vi "Main Archive and FTP 4_0.vi"() -> ()   [LabVIEW 2011]
doc: "FILE Archive & FTP is a software used to handle the file management of remote field sites using the HTI Data Logger or ATR series acoustic equipment that generates *.RAT and *.ATL files. The software monitors a specific folder on the local machine that the HTI equipment has been set up to move completed files of these types into. All other file types are ignored. The software continues to scan this file until a new file is added to the directory, on the addition of a file the NODE ARCHIVE & FTP software moves the file into an Archive directory (and if specified into a redundant Archive directory) then creates a *.ZIP version of the file and retains a copy of it in the Archive directory as well. All Zip files are then copied to a specified FTP host.\n\nNODE ARCHIVE & FTP will not try and move files for the last five minutes of an hour, or for the first five to ten minutes of the hour (based on CPU time). This is to allow the HTI hardware time to move all files at the top of the hour and avoid conflict. During the rest of the hour the software will continue to scan for new files. At any time a user can force a scan or FTP move by selecting the Manual Force FTP button or the Manual Archive Files button.\n\nNODE ARCHIVE & FTP creates an .INI file and a .CSV file in the programs application directory. The .INI file retains the last values of the file directory and FTP credentials used. The .CSV retains a history of *.ZIP files moved to the FTP and the status of their move, if there were errors or not. NODE ARCHIVE & FTP will continue to try and send the file to the FTP host until that file has completed the process with no errors. DO NOT remove or edit the .CSV file or the software will try and move all files up to the FTP again and will slow down the FTP Host."
uses:
  <vilib>/Utility/error.llb/DialogType.ctl
  <vilib>/Utility/sysdir.llb/System Directory Type.ctl
  Controls/FTP Credintials.ctl
  Controls/File Management.ctl
  Controls/File Path directories.ctl
  Controls/Ping address and email notify.ctl
panel:
  in  "ShutDown 2":bool
  in  "File type Cover 2":bool
  in  "Manual Archive 2":bool
  out "Email Notification Cluster":T1={"Mail Server"="", "Return Address"="", "Email User Name"="", "Password"="", "Ping Address 1"="10.0.0.40", "Ping Address 2"="google.com", "Ping Address FTP Host"="web1026.ixwebhosting.com", "Ping address 1"=FALSE, "Ping address 2"=FALSE, "Ping FTP Host"=FALSE}
  in  "shutting down closeout":bool
  in  "Time DaY":timestamp
  in  "Top level Tabs":T2(tab)
  in  "Auto Archive":bool
  in  "Auto FTP":bool
  in  "FTP Creds":T3 {"FTP Timeout (S)" min=0 max=300 step=1}
  in  "SITE ID":string="Site Not Configured" caption="Site ID:"
  in  "File Management":T4
  in  "Manual FTP":bool
  out "Archive in progress":bool caption="Archive"
  out "Status FTP move":bool caption="FTP"
  in  "Manual Archive":bool
  in  "File output directories":T5={"Archive Location"=path "", "Archive Location 2"=path "<Not A Path>", "OutPut Path"=path "", "Directory(s) To Scan Files"=[]}
  in  "Ping FTP Host":bool
  in  "Ping on Address 2":bool
  in  "Ping on Address 1":bool
  out "Response 2":bool
  in  "AddressNode2":string="www.google.com" caption="Ping Address for 2"
  out "FTP Host\nResponse":bool
  out "Response 1":bool
  in  "recipients":string[](array[string])=["nmswyers@gmail.com"] caption="Errors & Warnings Email Recipients"
  in  "Addresshost":string="50.6.185.144" caption="Ping Address of FTP"
  in  "AddressNode 1":string="10.0.0.40" caption="Ping Address for 1"
  out "Elapsed Time (H)":dbl caption="Time since Last File \nSize Check (H)" format="%#_3f"
  # "D\nI\nR\nE\nC\nT\nO\nR\nY\n\nS\nE\nT"
  # "FTP\n\nSETUP"
  # "FILE \n\nHANDLE\n\nMETHODS"
  # "File Handling Method"
  # "Addresses to Ping"
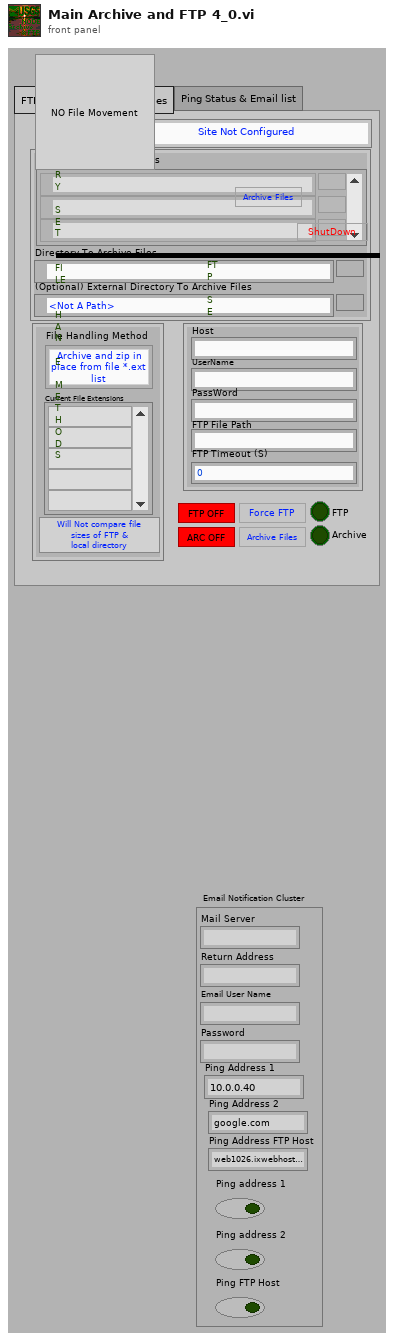
[diagram p1: front panel]
types:
  T1 = typedef "Ping address and email notify.ctl" = cluster{"Mail Server":string, "Return Address":string, "Email User Name":string, "Password":string, "Ping Address 1":string, "Ping Address 2":string, "Ping Address FTP Host":string, "Ping address 1":bool, "Ping address 2":bool, "Ping FTP Host":bool}
  T2 = enum32{"FTP Connection & Directories", "Ping Status & Email list"}
  T3 = typedef "FTP Credintials.ctl" = cluster{"Host":string, "UserName":string, "PassWord":string, "FTP File Path":string, "FTP Timeout (S)":i32, "Active or Passive":bool, "ASCII or Binary":bool}
  T4 = typedef "File Management.ctl" = cluster{"Comp File Size":bool, "File Handle Method":enum16{"Archive and zip in place from file *.ext list", "Archive and zip ALL file Types to archive directory", "Archive and zip to archive directory from file *.ext list", "Perform no file management"}, "file extention list":string[]}
  T5 = typedef "File Path directories.ctl" = cluster{"Archive Location":path, "Archive Location 2":path, "OutPut Path":path, "Directory(s) To Scan Files":path[]}
  T6 = enum16{"Archive and zip in place from file *.ext list", "Archive and zip ALL file Types to archive directory", "Archive and zip to archive directory from file *.ext list", "Perform no file management"}
  T7 = typedef "DialogType.ctl" = u16
  T8 = enum8{"Enabled", "Disabled", "Disabled and Grayed Out"}
  T9 = enum32{"invalid app kind", "Development System", "Run Time System", "Student Edition", "Embedded LabVIEW", "Evaluation", "Custom"}
  T10 = typedef "System Directory Type.ctl" = i32
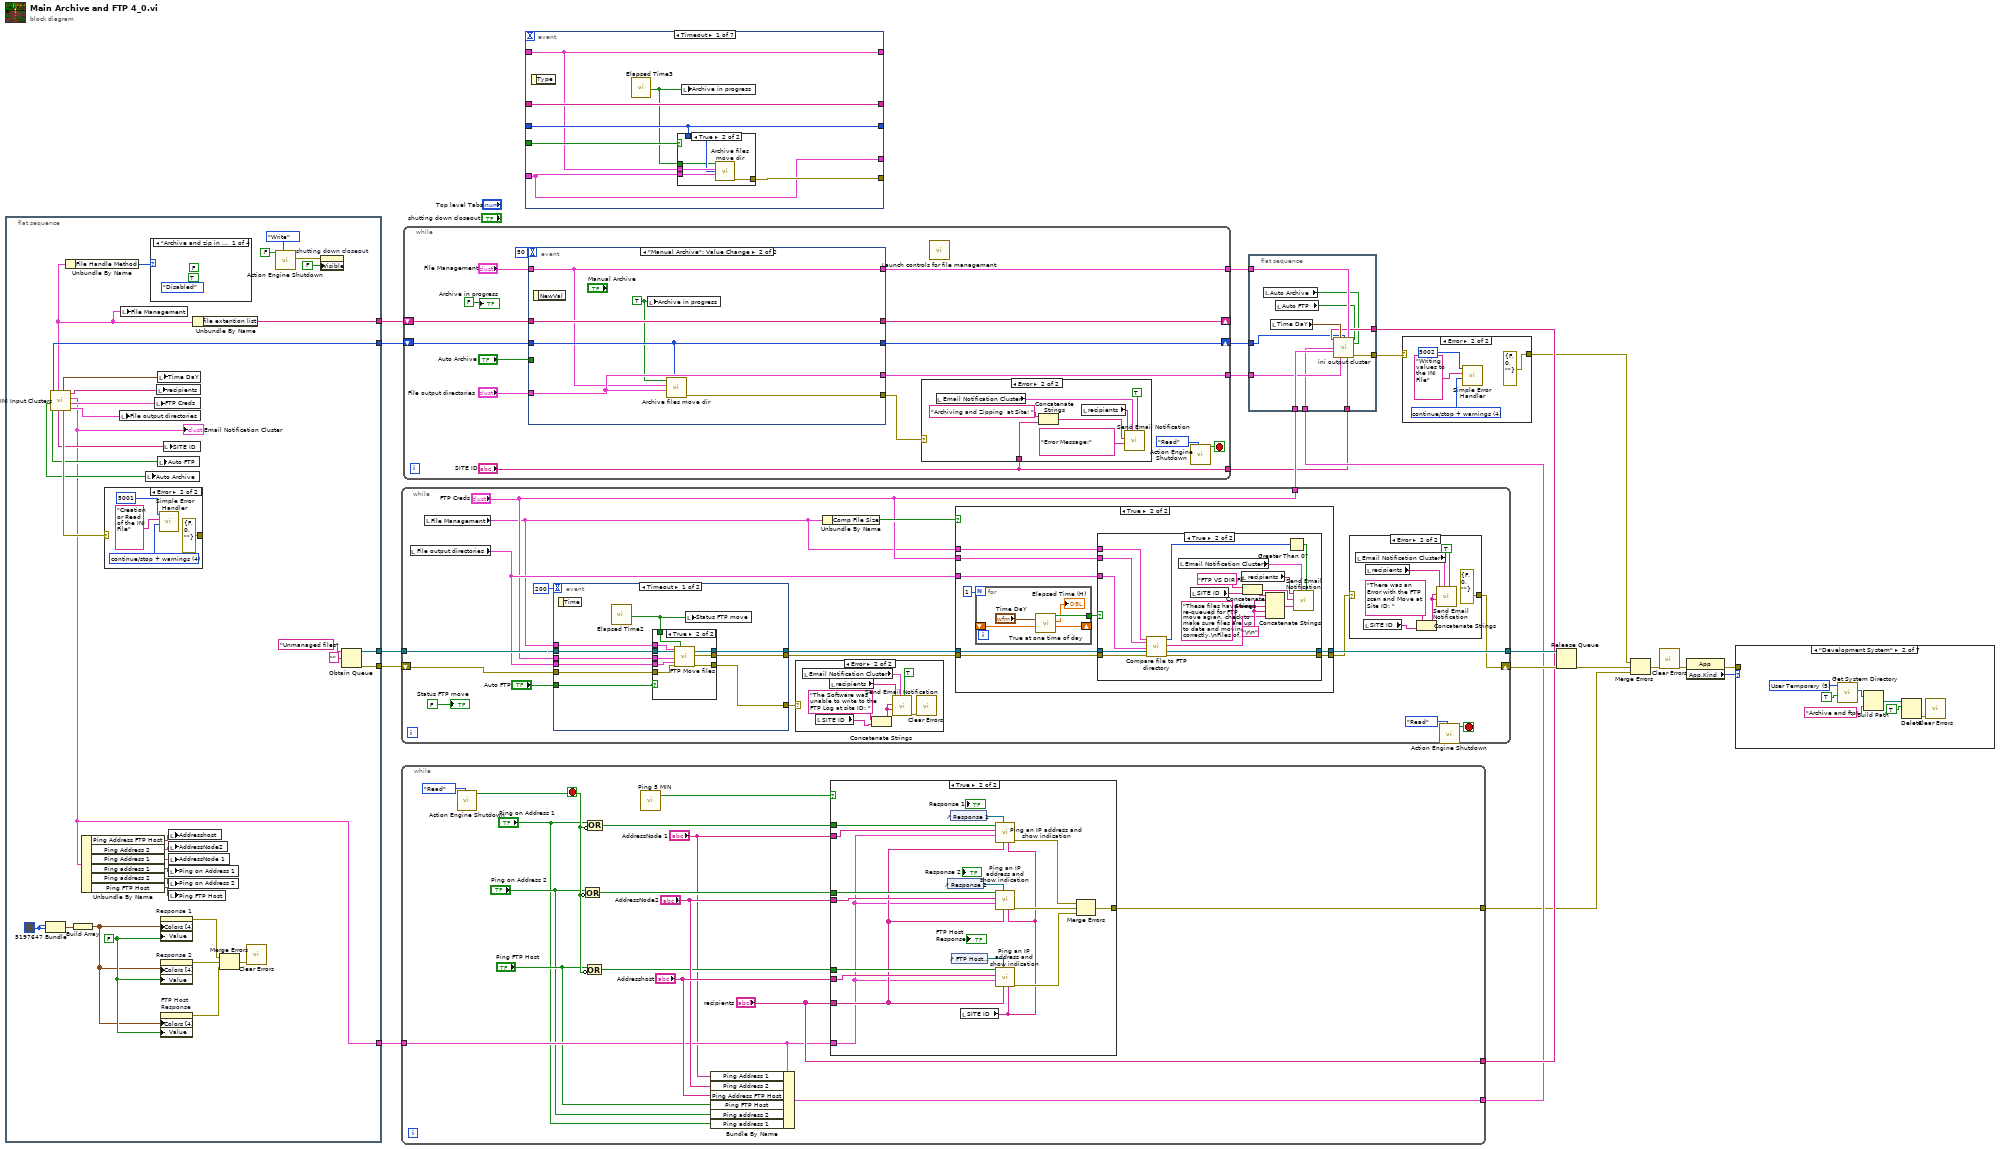
[diagram p0: block diagram]
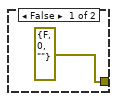
[diagram p2: hidden frame]
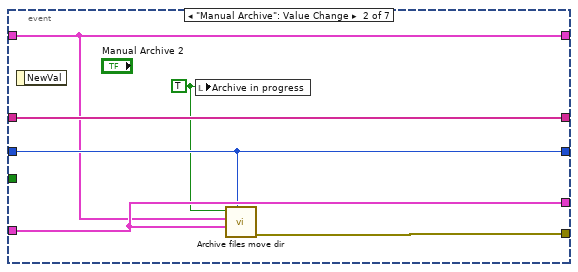
[diagram p3: hidden frame]
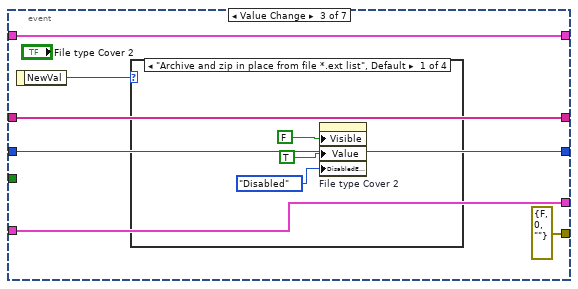
[diagram p4: hidden frame]
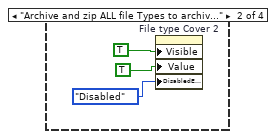
[diagram p5: hidden frame]
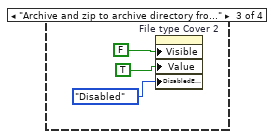
[diagram p6: hidden frame]
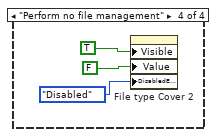
[diagram p7: hidden frame]
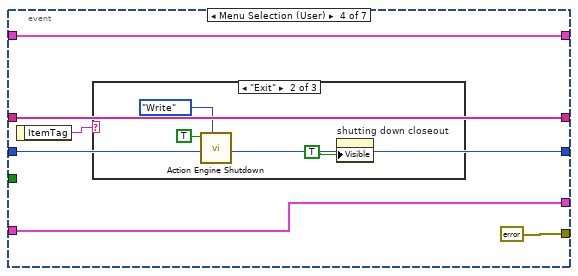
[diagram p8: hidden frame]
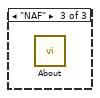
[diagram p10: hidden frame]
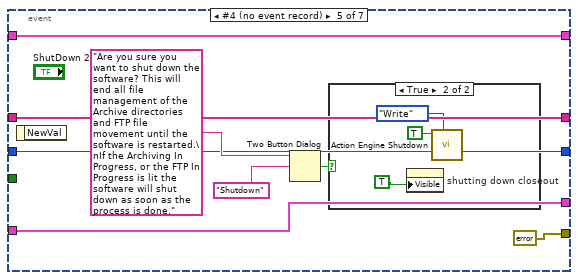
[diagram p11: hidden frame]
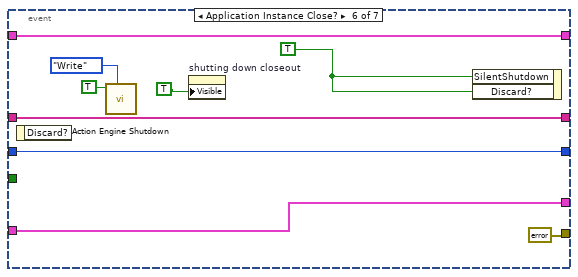
[diagram p13: hidden frame]
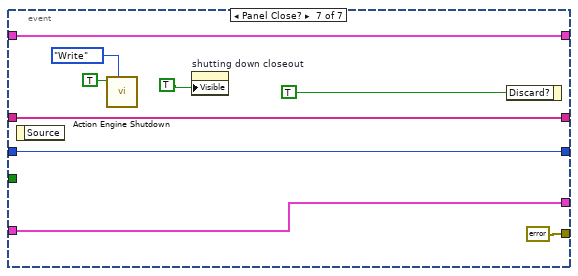
[diagram p14: hidden frame]
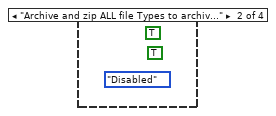
[diagram p15: hidden frame]
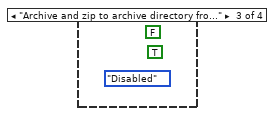
[diagram p16: hidden frame]
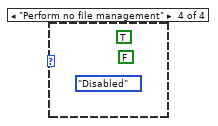
[diagram p17: hidden frame]
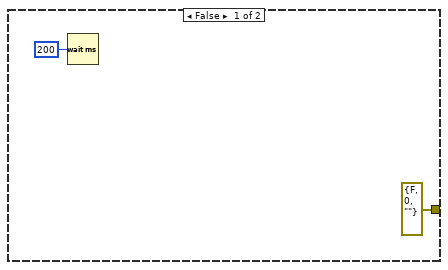
[diagram p19: hidden frame]
diagram:
  n1 = flat-sequence {
    tunnel: [w55] -> w22
    tunnel: [w54] -> w16
    tunnel: [w49] -> w15
    tunnel: [w45] -> w6
    tunnel: [w39] -> w3
    frame #0 {
      w26 = FALSE ("Response 1")
      w23 = u32 5197647 ("Color Box")
      n2 = Bundle("Color Box"=w23, "Color Box"=w23) -> (w24:cluster{"Color Box":u32, "Color Box":u32})  [unwired: 1 in]
      n3 = call "INI Input Clusters.vi"() -> ("File output directories"=w47:T5, "FTP CRED Cluster"=w50:T3, "Email Notification Cluster"=w39:T1, "Email Recipiant List"=w51:string[], "error out"=w53:errorcluster, "time stamp"=w52:timestamp, "Site ID"=w48:string, "File Management cluster"=w38:T4, "Auto FTP"=w41:bool, "Auto Archive"=w40:bool, "hours old date mod(hours)"=w45:u8)  [unwired: 1 in]
      "Email Notification Cluster" <- w39
      n4 = Unbundle By Name(w38) -> ("File Handle Method"=w37:T6)
      n5 = Build Array(w24) -> (w25:cluster{"Color Box":u32, "Color Box":u32}[])
      n6 = Unbundle By Name(w39) -> ("Ping Address FTP Host"=w36:string, "Ping Address 2"=w35:string, "Ping Address 1"=w34:string, "Ping address 1"=w33:bool, "Ping address 2"=w32:bool, "Ping FTP Host"=w31:bool)
      n7 = case shown="Error" w53 {
        selector: w53 -> [w66 _]
        tunnel: [w66 errorcluster {"status"=FALSE, "code"=0, "source"=""} ("error out")] -> _
        frame No Error {
        }
        frame Error {
          w70 = T7 4 items=["no dialog", "OK message", "continue or stop message", "OK message + warnings", "continue/stop + warnings"] ("type of dialog (OK msg:1)")
          n8 = call <vilib>:"Simple Error Handler.vi"("error code (no error:0)"=5001, "error source (\" \")"="Creation or Read of the INI File" ("error source (\" \")"), "type of dialog (OK msg:1)"=w70) -> ()  [unwired: 2 in, 5 out]
        }
      }
      n9 = local write "File output directories"(w47) -> ()
      n10 = local write "File Management"(w38) -> ()
      n11 = local write "Auto Archive"(w40) -> ()
      n12 = case shown="\"Archive and zip in place from file *.ext list\", Default" w37 {
        frame "Archive and zip in place from file *.ext list", Default {
          w58 = FALSE ("Visible")
          w59 = TRUE ("File type Cover")
          w60 = T8."Disabled" ("Disabled")
        }
        frame "Archive and zip ALL file Types to archive directory" {
          (unwired) TRUE ("Visible")
          (unwired) TRUE ("File type Cover")
          w61 = T8."Disabled" ("Disabled")
        }
        frame "Archive and zip to archive directory from file *.ext list" {
          (unwired) FALSE ("Visible")
          (unwired) TRUE ("File type Cover")
          w62 = T8."Disabled" ("Disabled")
        }
        frame "Perform no file management" {
          w63 = TRUE ("Visible")
          w64 = FALSE ("File type Cover")
          w65 = T8."Disabled" ("Disabled")
        }
      }
      n13 = local write "FTP Creds"(w50) -> ()
      n14 = local write "recipients"(w51) -> ()
      n15 = local write "Auto FTP"(w41) -> ()
      n16 = local write "Time DaY"(w52) -> ()
      n17 = property on="Response 1" class="Bool (strict)"("Colors [4]"=w25, "Value"=w26) -> (error out=w27:errorcluster)  [unwired: 2 in, 1 out]
      n18 = property on="Response 2" class="Bool (strict)"("Colors [4]"=w25, "Value"=w26) -> (error out=w28:errorcluster)  [unwired: 2 in, 1 out]
      n19 = property on="FTP Host\nResponse" class="Bool (strict)"("Colors [4]"=w25, "Value"=w26) -> (error out=w29:errorcluster)  [unwired: 2 in, 1 out]
      n20 = local write "SITE ID"(w48) -> ()
      n21 = local write "Addresshost"(w36) -> ()
      n22 = local write "AddressNode2"(w35) -> ()
      n23 = local write "AddressNode 1"(w34) -> ()
      n24 = local write "Ping on Address 1"(w33) -> ()
      n25 = local write "Ping on Address 2"(w32) -> ()
      n26 = local write "Ping FTP Host"(w31) -> ()
      n27 = Unbundle By Name(w38) -> ("file extention list"=w49:string[])
      n28 = Merge Errors(w27, w28, w29) -> (w30:errorcluster)
      n29 = call <vilib>:"Clear Errors.vi"("error in (no error)"=w30) -> ()  [unwired: 6 in, 1 out]
      n30 = call "Action Engine Shutdown.vi"("Shutdown"=enum16{"Write", "Read"}."Write", "Shutdown (True to Shutdown)"=FALSE) -> ("error out"=w42:errorcluster)  [unwired: 8 in, 1 out]
      n31 = property on="shutting down closeout" class="Bool"(error in=w42, "Visible"=FALSE) -> ()  [unwired: 1 in, 2 out]
      n32 = Obtain Queue(name (unnamed)="Unmanaged files", element data type="" ("name (unnamed)")) -> (queue out=w55:refnum<queue>, error out=w54:errorcluster)  [unwired: 3 in, 1 out]
    }
  }
  n33 = while {
    tunnel: w22 -> [w86]
    tunnel: [w84] -> w20
    tunnel: ["FTP Creds"] -> w12
    shift-right: [w82] -> w17
    shift-left: w16 -> [w81]
    stop <- w72 stop-if-true
    n34 = local read "File output directories"() -> (w76:T5)
    n35 = local read "File Management"() -> (w74:T4)
    n36 = event shown="[0] Timeout" {
      selector: _ -> [_ _]
      dyn-events: _ -> [_ _]
      timeout: 200 -> [_ _]
      tunnel: w86 -> [w148 w165]
      tunnel: [w147 w166] -> w85
      tunnel: w81 -> [w146 w162]
      tunnel: [w145 w167] -> w83
      tunnel: [w144 w168] -> w79
      tunnel: "FTP Creds" -> [w143 w164]
      tunnel: w76 -> [w141 w161]
      tunnel: w74 -> [w142 w163]
      tunnel: "Auto FTP" -> [w140 _]
      event Timeout {
        n37 = event-data() -> ()  [unwired: 1 in, 1 out]
        n38 = call "Elapsed Time2"() -> ("Time has Elapsed"=w139:bool)  [unwired: 12 in, 7 out]
        n39 = case shown="True" w140 {
          tunnel: w139 -> [_ w160]
          tunnel: [w151 w159] -> w147
          tunnel: [errorcluster {"status"=FALSE, "code"=0, "source"=""} ("Log file write error condition") w158] -> w144
          tunnel: [w150 w157] -> w145
          tunnel: w148 -> [w151 w156]
          tunnel: w142 -> [_ w155]
          tunnel: w146 -> [w150 w153]
          tunnel: w143 -> [_ w154]
          tunnel: w141 -> [_ w152]
          frame False {
          }
          frame True {
            n40 = call "FTP Move files.vi"("File Management"=w155, "Unmanaged Files Queue"=w156, "FTP Creds"=w154, "File output directories"=w152, "Unmanaged Files prior errors"=w153, "Timing true or false to zip files"=w160) -> ("Unmanaged Files Queue out"=w159:refnum<queue>, "Unmanaged files queue error out"=w157:errorcluster, "Log file write error condition"=w158:errorcluster)  [unwired: 11 in]
          }
        }
        n41 = local write "Status FTP move"(w139) -> ()
      }
      event "Manual FTP": Value Change {
        n42 = event-data() -> ()  [unwired: 1 in, 1 out]
        n43 = call "FTP Move files.vi"("File Management"=w163, "Unmanaged Files Queue"=w165, "FTP Creds"=w164, "File output directories"=w161, "Unmanaged Files prior errors"=w162, "Timing true or false to zip files"=TRUE) -> ("Unmanaged Files Queue out"=w166:refnum<queue>, "Unmanaged files queue error out"=w167:errorcluster, "Log file write error condition"=w168:errorcluster)  [unwired: 11 in]
        n44 = local write "Status FTP move"(TRUE ("Status FTP move")) -> ()
      }
    }
    n45 = case shown="Error" w79 {
      frame No Error {
      }
      frame Error {
        n46 = local read "Email Notification Cluster"() -> (w89:T1)
        n47 = local read "SITE ID"() -> (w90:string)
        n48 = local read "recipients"() -> (w94:string[])
        n49 = Concatenate Strings("The Software was unable to write to the FTP Log at site ID: " ("Email Subject"), w90) -> (w91:string)
        n50 = call "Send Email Notification.vi"("Send Email Notification"=TRUE, "Email Notification Cluster (in)"=w89, "message"=w91, "Email Subject"=w91, "recipients"=w94) -> ("error out"=w88:errorcluster)  [unwired: 6 in]
        n51 = call <vilib>:"Clear Errors.vi"("error in (no error)"=w88) -> ()  [unwired: 6 in, 1 out]
      }
    }
    n52 = Unbundle By Name(w74) -> ("Comp File Size"=w77:bool)
    n53 = case shown="True" w77 {
      tunnel: w85 -> [w104 w112]
      tunnel: [w104 w111] -> w84
      tunnel: w83 -> [w103 w109]
      tunnel: [w103 w110] -> w80
      tunnel: "FTP Creds" -> [_ w108]
      tunnel: w76 -> [_ w106]
      tunnel: w74 -> [_ w105]
      frame False {
      }
      frame True {
        n54 = for {
          N: 1 -> [_]
          tunnel: [w117] -> w113
          shift-right: [w115] -> _
          shift-left: _ -> [w114]
          n55 = call "True at one time of day.vi"("Next start time in"=w114, "Time stamp from INI (only will use time Not date)"="Time DaY") -> ("next start time out"=w115:dbl, "Time Until Next Scan (H)"=→"Elapsed Time (H)":dbl, "Time has Elapsed"=w117:bool)  [unwired: 6 in, 1 out]
        }
        n56 = case shown="True" w113 {
          tunnel: w112 -> [w120 w128]
          tunnel: [w120 w129] -> w111
          tunnel: [w119 w127] -> w110
          tunnel: w109 -> [w119 w130]
          tunnel: w108 -> [_ w124]
          tunnel: w106 -> [_ w123]
          tunnel: w105 -> [_ w122]
          frame False {
          }
          frame True {
            w136 = "\r\n"
            n57 = call "Compare file to FTP directory.vi"("File Management"=w122, "FTP Creds"=w124, "File output directories"=w123, "Unmanaged Files Queue"=w128, "Unmanaged files queue error"=w130) -> ("number of unmached files"=w126:i32, "unmatched file names"=w125:string, "Unmanaged Files Queue out"=w129:refnum<queue>, "Unmanaged files queue error out"=w127:errorcluster)  [unwired: 11 in]
            n58 = local read "Email Notification Cluster"() -> (w121:T1)
            n59 = local read "SITE ID"() -> (w131:string)
            n60 = local read "recipients"() -> (w134:string[])
            n61 = Concatenate Strings("FTP VS DIR File sizes are different at Site ID: " ("string"), w131) -> (w133:string)
            n62 = Concatenate Strings(w133, w136, "These files have been re-queued for FTP move agian, check to make sure files are up to date and moving correctly.\nFiles of issue are listed below.\n\nLIST:" ("string"), w136, w125) -> (w132:string)
            n63 = Greater Than 0?(x=w126) -> (x > 0?=w135:bool)
            n64 = call "Send Email Notification.vi"("Send Email Notification"=w135, "Email Notification Cluster (in)"=w121, "message"=w132, "Email Subject"=w133, "recipients"=w134) -> ()  [unwired: 6 in, 1 out]
          }
        }
      }
    }
    n65 = case shown="Error" w80 {
      selector: w80 -> [w95 _]
      tunnel: [w95 errorcluster {"status"=FALSE, "code"=0, "source"=""} ("error IO")] -> w82
      frame No Error {
      }
      frame Error {
        n66 = local read "Email Notification Cluster"() -> (w96:T1)
        n67 = local read "SITE ID"() -> (w97:string)
        n68 = local read "recipients"() -> (w101:string[])
        n69 = Concatenate Strings("There was an Error with the FTP scan and Move at Site ID: " ("Email Subject"), w97) -> (w98:string)
        n70 = call "Send Email Notification.vi"("Send Email Notification"=TRUE, "Email Notification Cluster (in)"=w96, "message"=w98, "Email Subject"=w98, "recipients"=w101) -> ()  [unwired: 6 in, 1 out]
      }
    }
    n71 = call "Action Engine Shutdown.vi"("Shutdown"=enum16{"Write", "Read"}."Read") -> ("Shutdown"=w72:bool)  [unwired: 9 in, 1 out]
    "Status FTP move" <- FALSE ("Status FTP move")
  }
  n72 = while {
    tunnel: w3 -> [w178]
    tunnel: [w184] -> w9
    tunnel: ["recipients"] -> w10
    tunnel: [w171] -> w2
    stop <- w176 stop-if-true
    n73 = call "Action Engine Shutdown.vi"("Shutdown"=enum16{"Write", "Read"}."Read") -> ("Shutdown"=w176:bool)  [unwired: 9 in, 1 out]
    n74 = Compound Arithmetic op=OR("Ping on Address 2", invert w176) -> (w182:bool)
    n75 = Compound Arithmetic op=OR("Ping FTP Host", invert w176) -> (w181:bool)
    n76 = Compound Arithmetic op=OR("Ping on Address 1", invert w176) -> (w183:bool)
    n77 = call "Ping 5 MIN"() -> ("Time has Elapsed"=w180:bool)  [unwired: 12 in, 7 out]
    n78 = Bundle By Name(cluster=w178, "Ping Address 1"="AddressNode 1", "Ping Address 2"="AddressNode2", "Ping Address FTP Host"="Addresshost", "Ping FTP Host"="Ping FTP Host", "Ping address 2"="Ping on Address 2", "Ping address 1"="Ping on Address 1") -> (w184:T1)
    n79 = case shown="True" w180 {
      tunnel: "recipients" -> [_ w190]
      tunnel: w178 -> [_ w189]
      tunnel: "Addresshost" -> [_ w196]
      tunnel: "AddressNode2" -> [_ w197]
      tunnel: "AddressNode 1" -> [_ w204]
      tunnel: w183 -> [_ w202]
      tunnel: w182 -> [_ w200]
      tunnel: w181 -> [_ w198]
      tunnel: [errorcluster {"status"=FALSE, "code"=0, "source"=""} ("error IO") w195] -> w171
      frame False {
        n80 = Wait (ms)(milliseconds to wait=u32 200) -> ()  [unwired: 1 out]
      }
      frame True {
        n81 = control-ref of="Response 2"() -> (w201:refnum<vi>)
        n82 = control-ref of="Response 1"() -> (w203:refnum<vi>)
        n83 = control-ref of="FTP Host\nResponse"() -> (w199:refnum<vi>)
        n84 = local read "SITE ID"() -> (w191:string)
        n85 = call "Ping an IP address and show indication.vi"("SITE ID"=w191, "recipients"=w190, "Responce Lite Reference"=w203, "Email Notification Cluster"=w189, "AddressNode 1"=w204, "Ping Site"=w202) -> ("error out"=w194:errorcluster)  [unwired: 5 in]
        n86 = call "Ping an IP address and show indication.vi"("SITE ID"=w191, "recipients"=w190, "Responce Lite Reference"=w201, "Email Notification Cluster"=w189, "AddressNode 1"=w197, "Ping Site"=w200) -> ("error out"=w193:errorcluster)  [unwired: 5 in]
        n87 = call "Ping an IP address and show indication.vi"("SITE ID"=w191, "recipients"=w190, "Responce Lite Reference"=w199, "Email Notification Cluster"=w189, "AddressNode 1"=w196, "Ping Site"=w198) -> ("error out"=w192:errorcluster)  [unwired: 5 in]
        n88 = Merge Errors(w194, w193, w192) -> (w195:errorcluster)
      }
    }
  }
  n89 = while {
    tunnel: [w216] -> w11
    shift-right: [w212] -> _
    shift-left: w15 -> [w217]
    tunnel: [w211] -> w13
    tunnel: ["SITE ID"] -> w8
    shift-right: [w209] -> w7
    shift-left: w6 -> [w210]
    stop <- w207 stop-if-true
    n90 = event shown="[1] \"Manual Archive\": Value Change" {
      selector: _ -> [_ _]
      dyn-events: _ -> [_ _]
      timeout: 50 -> [_ _]
      tunnel: [w233 w245] -> w206
      tunnel: w217 -> [w231 w243]
      tunnel: "File output directories" -> [w232 w244]
      tunnel: [w232 w244] -> w216
      tunnel: [w228 w240] -> w211
      tunnel: "File Management" -> [w228 w240]
      tunnel: [w231 w243] -> w212
      tunnel: w210 -> [w230 w242]
      tunnel: [w230 w242] -> w209
      tunnel: "Auto Archive" -> [w229 _]
      event Timeout {
        n91 = event-data() -> ()  [unwired: 1 in, 1 out]
        n92 = call "Elapsed Time"() -> ("Time has Elapsed"=w227:bool)  [unwired: 12 in, 7 out]
        n93 = case shown="True" w229 {
          tunnel: w232 -> [_ w239]
          tunnel: [errorcluster {"status"=FALSE, "code"=0, "source"=""} ("error IO") w238] -> w233
          tunnel: w228 -> [_ w237]
          tunnel: w230 -> [_ w236]
          tunnel: w227 -> [_ w235]
          frame False {
          }
          frame True {
            n94 = call "Archive files move dir.vi"("hours old date mod(hours)"=w236, "File path input cluster"=w239, "File Management"=w237, "Timing True to archive"=w235) -> ("error IO"=w238:errorcluster)  [unwired: 5 in]
          }
        }
        n95 = local write "Archive in progress"(w227) -> ()
      }
      event "Manual Archive": Value Change {
        w241 = TRUE ("Status File move")
        n96 = event-data() -> ()  [unwired: 1 in, 1 out]
        n97 = local write "Archive in progress"(w241) -> ()
        n98 = call "Archive files move dir.vi"("hours old date mod(hours)"=w242, "File path input cluster"=w244, "File Management"=w240, "Timing True to archive"=w241) -> ("error IO"=w245:errorcluster)  [unwired: 5 in]
      }
    }
    n99 = case shown="Error" w206 {
      tunnel: "SITE ID" -> [_ w222]
      frame No Error {
      }
      frame Error {
        n100 = local read "Email Notification Cluster"() -> (w220:T1)
        n101 = Concatenate Strings("Archiving and Zipping  at Site: " ("Email Subject"), w222) -> (w223:string)
        n102 = local read "recipients"() -> (w226:string[])
        n103 = call "Send Email Notification.vi"("Send Email Notification"=TRUE, "Email Notification Cluster (in)"=w220, "message"="Error Message:", "Email Subject"=w223, "recipients"=w226) -> ()  [unwired: 6 in, 1 out]
      }
    }
    n104 = call "Launch controls for file management.vi"() -> ()  [unwired: 10 in, 2 out]
    n105 = call "Action Engine Shutdown.vi"("Shutdown"=enum16{"Write", "Read"}."Read") -> ("Shutdown"=w207:bool)  [unwired: 9 in, 1 out]
    "Archive in progress" <- FALSE ("Archive in progress")
  }
  n106 = event shown="[0] Timeout" {
    selector: _ -> [_ _ _ _ _ _ _]
    dyn-events: _ -> [_ _ _ _ _ _ _]
    timeout: _ -> [_ _ _ _ _ _ _]
    tunnel: [w252 w264 errorcluster {"status"=FALSE, "code"=0, "source"=""} ("error IO") errorcluster {"status"=FALSE, "code"=0, "source"=""} ("error IO") errorcluster {"status"=FALSE, "code"=0, "source"=""} ("error IO") errorcluster {"status"=FALSE, "code"=0, "source"=""} ("error IO") errorcluster {"status"=FALSE, "code"=0, "source"=""} ("error IO")] -> _
    tunnel: _ -> [w250 w262 w268 w284 w295 w306 w315]
    tunnel: _ -> [w251 w263 w270 w287 w293 w304 w313]
    tunnel: [w251 w263 w270 w287 w293 w304 w313] -> _
    tunnel: [w247 w259 w269 w286 w296 w307 w316] -> _
    tunnel: _ -> [w247 w259 w269 w286 w296 w307 w316]
    tunnel: [w250 w262 w268 w284 w295 w306 w315] -> _
    tunnel: _ -> [w249 w261 w267 w285 w294 w305 w314]
    tunnel: [w249 w261 w267 w285 w294 w305 w314] -> _
    tunnel: _ -> [w248 _ _ _ _ _ _]
    event Timeout {
      n107 = event-data() -> ()  [unwired: 1 in, 1 out]
      n108 = call "Elapsed Time3"() -> ("Time has Elapsed"=w246:bool)  [unwired: 12 in, 7 out]
      n109 = case shown="True" w248 {
        tunnel: w251 -> [_ w258]
        tunnel: [errorcluster {"status"=FALSE, "code"=0, "source"=""} ("error IO") w257] -> w252
        tunnel: w247 -> [_ w256]
        tunnel: w249 -> [_ w255]
        tunnel: w246 -> [_ w254]
        frame False {
        }
        frame True {
          n110 = call "Archive files move dir.vi"("hours old date mod(hours)"=w255, "File path input cluster"=w258, "File Management"=w256, "Timing True to archive"=w254) -> ("error IO"=w257:errorcluster)  [unwired: 5 in]
        }
      }
      n111 = local write "Archive in progress"(w246) -> ()
    }
    event "Manual Archive": Value Change {
      w260 = TRUE ("Status File move")
      n112 = event-data() -> ()  [unwired: 1 in, 1 out]
      n113 = local write "Archive in progress"(w260) -> ()
      n114 = call "Archive files move dir.vi"("hours old date mod(hours)"=w261, "File path input cluster"=w263, "File Management"=w259, "Timing True to archive"=w260) -> ("error IO"=w264:errorcluster)  [unwired: 5 in]
    }
    event Value Change {
      n115 = event-data() -> ("NewVal"=w266:T6)  [unwired: 1 in]
      n116 = case shown="\"Archive and zip in place from file *.ext list\", Default" w266 {
        frame "Archive and zip in place from file *.ext list", Default {
          n117 = property on="File type Cover 2" class="Bool (strict)"("Visible"=FALSE, "Value"=TRUE ("File type Cover"), "DisabledEnum"=T8."Disabled" ("Disabled")) -> ()  [unwired: 2 in, 2 out]
        }
        frame "Archive and zip ALL file Types to archive directory" {
          n118 = property on="File type Cover 2" class="Bool (strict)"("Visible"=TRUE, "Value"=TRUE ("File type Cover"), "DisabledEnum"=T8."Disabled" ("Disabled")) -> ()  [unwired: 2 in, 2 out]
        }
        frame "Archive and zip to archive directory from file *.ext list" {
          n119 = property on="File type Cover 2" class="Bool (strict)"("Visible"=FALSE, "Value"=TRUE ("File type Cover"), "DisabledEnum"=T8."Disabled" ("Disabled")) -> ()  [unwired: 2 in, 2 out]
        }
        frame "Perform no file management" {
          n120 = property on="File type Cover 2" class="Bool (strict)"("Visible"=TRUE, "Value"=FALSE ("File type Cover"), "DisabledEnum"=T8."Disabled" ("Disabled")) -> ()  [unwired: 2 in, 2 out]
        }
      }
    }
    event Menu Selection (User) {
      n121 = event-data() -> ("ItemTag"=w288:string)  [unwired: 1 in]
      n122 = case shown="\"Exit\"" w288 {
        frame "Null", Default {
        }
        frame "Exit" {
          n123 = call "Action Engine Shutdown.vi"("Shutdown"=enum16{"Write", "Read"}."Write", "Shutdown (True to Shutdown)"=TRUE ("Stop Button")) -> ()  [unwired: 8 in, 2 out]
          n124 = property on="shutting down closeout" class="Bool"("Visible"=TRUE) -> ()  [unwired: 2 in, 2 out]
        }
        frame "NAF" {
          n125 = call "About.vi"() -> ()  [unwired: 12 in]
        }
      }
    }
    event #4 (no event record) {
      n126 = event-data() -> ()  [unwired: 1 in, 1 out]
      n127 = Two Button Dialog(message="Are you sure you want to shut down the software? This will end all file management of the Archive directories and FTP file movement until the software is restarted.\nIf the Archiving In Progress, or the FTP In Progress is lit the software will shut down as soon as the process is done.", 2:"Shutdown" ("T button name (\"OK\")")) -> (T button?=w299:bool)  [unwired: 1 in]
      n128 = case shown="True" w299 {
        frame False {
        }
        frame True {
          n129 = property on="shutting down closeout" class="Bool"("Visible"=TRUE) -> ()  [unwired: 2 in, 2 out]
          n130 = call "Action Engine Shutdown.vi"("Shutdown"=enum16{"Write", "Read"}."Write", "Shutdown (True to Shutdown)"=TRUE) -> ()  [unwired: 8 in, 2 out]
        }
      }
    }
    event Application Instance Close? {
      w311 = TRUE ("SilentShutdown")
      n131 = event-data() -> ()  [unwired: 1 in, 1 out]
      n132 = call "Action Engine Shutdown.vi"("Shutdown"=enum16{"Write", "Read"}."Write", "Shutdown (True to Shutdown)"=TRUE) -> ()  [unwired: 8 in, 2 out]
      n133 = property on="shutting down closeout" class="Bool"("Visible"=TRUE) -> ()  [unwired: 2 in, 2 out]
      n134 = event-data("SilentShutdown"=w311, "Discard?"=w311) -> ()  [unwired: 1 in, 1 out]
    }
    event Panel Close? {
      n135 = event-data() -> ()  [unwired: 1 in, 1 out]
      n136 = call "Action Engine Shutdown.vi"("Shutdown"=enum16{"Write", "Read"}."Write", "Shutdown (True to Shutdown)"=TRUE) -> ()  [unwired: 8 in, 2 out]
      n137 = property on="shutting down closeout" class="Bool"("Visible"=TRUE) -> ()  [unwired: 2 in, 2 out]
      n138 = event-data("Discard?"=TRUE) -> ()  [unwired: 1 in, 1 out]
    }
  }
  n139 = flat-sequence {
    tunnel: [w331] -> w14
    tunnel: w13 -> [w329]
    tunnel: w12 -> [w328]
    tunnel: w11 -> [w327]
    tunnel: w10 -> [w326]
    tunnel: w9 -> [w321]
    tunnel: w8 -> [w325]
    tunnel: w7 -> [w324]
    frame #0 {
      n140 = local read "Auto Archive"() -> (w322:bool)
      n141 = local read "Time DaY"() -> (w330:timestamp)
      n142 = local read "Auto FTP"() -> (w323:bool)
      n143 = call "ini output cluster.vi"("recipients"=w326, "time stamp"=w330, "hours old date mod(hours)"=w324, "File Management"=w329, "Auto FTP"=w323, "Auto Archive"=w322, "Email Notification Cluster"=w321, "FTP Creds"=w328, "File Path Cluster"=w327, "SITE ID"=w325) -> ("error out"=w331:errorcluster)  [unwired: 5 in]
    }
  }
  n144 = case shown="Error" w14 {
    selector: w14 -> [w332 _]
    tunnel: [w332 errorcluster {"status"=FALSE, "code"=0, "source"=""} ("error IO")] -> w5
    frame No Error {
    }
    frame Error {
      w336 = T7 4 items=["no dialog", "OK message", "continue or stop message", "OK message + warnings", "continue/stop + warnings"] ("type of dialog (OK msg:1)")
      n145 = call <vilib>:"Simple Error Handler.vi"("error code (no error:0)"=5002, "error source (\" \")"="Writing values to the INI File" ("error source (\" \")"), "type of dialog (OK msg:1)"=w336) -> ()  [unwired: 2 in, 5 out]
    }
  }
  n146 = Release Queue(queue=w20, error in (no error)=w17) -> (error out=w1:errorcluster)  [unwired: 1 in, 2 out]
  n147 = Merge Errors(w5, w1, w2) -> (w4:errorcluster)
  n148 = call <vilib>:"Clear Errors.vi"("error in (no error)"=w4) -> ("error out"=w18:errorcluster)  [unwired: 6 in]
  n149 = property class="App"(error in=w18) -> (error out=w19:errorcluster, "App.Kind"=w21:T9)  [unwired: 1 in, 1 out]
  n150 = case shown="\"Development System\"" w21 {
    tunnel: w19 -> [_ _ _ _ _ _ _]
    frame "invalid app kind", Default {
    }
    frame "Development System" {
      w338 = T10 5 items=["User Home"=0, "User Desktop"=1, "User Documents"=2, "User Application Data"=3, "User Preferences"=4, "User Temporary"=5, "Public Documents"=6, "Public Application Data"=7, "Public Preferences"=8, "Public Cache"=13, "System Core Libraries"=9, "System Installed Libraries"=10, "Application Files"=11, "Boot Volume Root"=12] ("system directory type")
      n151 = call <vilib>:"Get System Directory.vi"("create directory if not found? (F)"=TRUE, "system directory type"=w338) -> ("system directory"=w340:path)  [unwired: 9 in]
      n152 = Build Path(base path=w340, name or relative path="Archive and ftp") -> (appended path=w342:path)
      n153 = Delete(path (use dialog)=w342, entire hierarchy (F)=TRUE) -> (error out=w337:errorcluster)  [unwired: 3 in, 2 out]
      n154 = call <vilib>:"Clear Errors.vi"("error in (no error)"=w337) -> ()  [unwired: 6 in, 1 out]
    }
    frame "Run Time System" {
      n155 = flat-sequence {
        frame #0 {
          w345 = T10 5 items=["User Home"=0, "User Desktop"=1, "User Documents"=2, "User Application Data"=3, "User Preferences"=4, "User Temporary"=5, "Public Documents"=6, "Public Application Data"=7, "Public Preferences"=8, "Public Cache"=13, "System Core Libraries"=9, "System Installed Libraries"=10, "Application Files"=11, "Boot Volume Root"=12] ("system directory type")
          n156 = call <vilib>:"Get System Directory.vi"("create directory if not found? (F)"=TRUE, "system directory type"=w345) -> ("system directory"=w347:path)  [unwired: 9 in]
          n157 = Build Path(base path=w347, name or relative path="Archive and ftp") -> (appended path=w349:path)
          n158 = Delete(path (use dialog)=w349, entire hierarchy (F)=TRUE) -> (error out=w344:errorcluster)  [unwired: 3 in, 2 out]
          n159 = call <vilib>:"Clear Errors.vi"("error in (no error)"=w344) -> ()  [unwired: 6 in, 1 out]
        }
        frame #1 {
          n160 = Quit LabVIEW() -> ()  [unwired: 1 in]
        }
      }
    }
    frame "Student Edition" {
    }
    frame "Embedded LabVIEW" {
    }
    frame "Evaluation" {
    }
    frame "Custom" {
    }
  }
